vi "Drive.vi"(11 "CTR to CMNDS":T1) -> ()   [LabVIEW 2014]
uses:
  JoyStick/Commands.ctl
  Global Variables/Refnums.vi
  <vilib>/Rock Robotics/WPI/RobotDrive/WPI_RobotDriveGetSetRefNum.vi
  <vilib>/Rock Robotics/WPI/RobotDrive/WPI_RobotDriveArcadeDrive_Standard(NoSaturation).vi
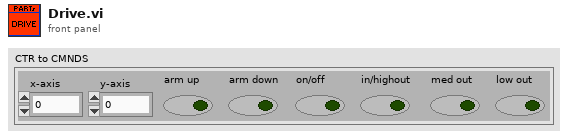
[diagram p1: front panel]
types:
  T1 = typedef "Commands.ctl" = cluster{"x-axis":dbl, "y-axis":dbl, "arm up":bool, "arm down":bool, "on/off":bool, "in/highout":bool, "med out":bool, "low out":bool}
  T2 = typedef "WPI_RobotDriveDevRef.ctl" = cluster{"DevStatus":errorcluster, "Motors[]":T3[], "Square Inputs":bool, "Max Output":dbl}
  T3 = typedef "WPI_MotorControlDeviceRef.ctl" = cluster{"DeviceStatus":errorcluster, "Type":enum16{"PWM", "CAN"}, "PWM":cluster{"Digital Module":T4, "PWM Channel":T5, "DeadBand":T6}, "CAN":cluster{"Device Number":u8, "Control Mode":T7, "Semaphore":T8, "Max Vout":dbl}, "Invert":bool, "TransformRef":T9, "InvTransformRef":T9}
  T4 = typedef "FPGA_TypedefDigitalModule.ctl" = enum16{"Digital Module 1", "Digital Module 2"}
  T5 = typedef "FPGA_DIOPWMChannel.ctl" = enum8{"PWM 1", "PWM 2", "PWM 3", "PWM 4", "PWM 5", "PWM 6", "PWM 7", "PWM 8", "PWM 9", "PWM 10", "Invalid"}
  T6 = typedef "WPI_PWMDeadband.ctl" = cluster{"Name":string, "maxPositivePwm":i32, "minPositivePwm":i32, "centerPwm":i32, "maxNegativePwm":i32, "minNegativePwm":i32, "angularRange":u16}
  T7 = typedef "WPI_CANJaguar_ControlMode.ctl" = enum8{"Percent VBus", "Current", "Speed", "Position", "Voltage"}
  T8 = typedef "Semaphore RefNum" = refnum<k1>
  T9 = typedef "WPI_PWMTransform_ConPane.ctl" = refnum<vi>
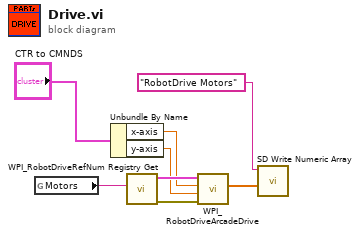
[diagram p0: block diagram]
diagram:
  n1 = global read "Refnums.vi" "Motors"() -> (w5:string)
  n2 = Unbundle By Name("CTR to CMNDS") -> ("x-axis"=w2:dbl, "y-axis"=w3:dbl)
  n3 = call <vilib>:"WPI_RobotDriveRefNum Registry Get.vi"("refnum name"=w5) -> ("error out"=w6:errorcluster, "RobotDriveDevRef"=w7:T2)  [unwired: 9 in]
  n4 = call-poly <vilib>:"WPI_RobotDriveArcadeDrive.vi"("error in (no error)"=w6, "Y axis value"=w3, "X axis value"=w2, "RobotDriveDevRef"=w7) -> ("Motor Values"=w1:dbl[])  [unwired: 5 in, 2 out]
  n5 = call <vilib>:"SD Write Numeric Array.vi"("Numeric Array"=w1, "Name"="RobotDrive Motors") -> ()  [unwired: 8 in, 2 out]
